vi "SRV_PM_Data Byte Unstuffing.vi"(0 "Stuffed Data":u8[](array[numeric]) format="%.0x", 1 "Data Length":u32, 11 "error in (no error)":errorcluster) -> (4 "Stuffed Data dup":u8[](array[numeric]) format="%.0x", 8 "Data":u8[](array[numeric]) format="%.0x", 10 "All Data Received?":bool, 14 "Remaining Stuffed Data":u8[](array[numeric]) format="%.0x", 15 "error out":errorcluster)   [LabVIEW 2009]
panel:
  in  "Stuffing Byte (0x00)":u8 format="%.0x"
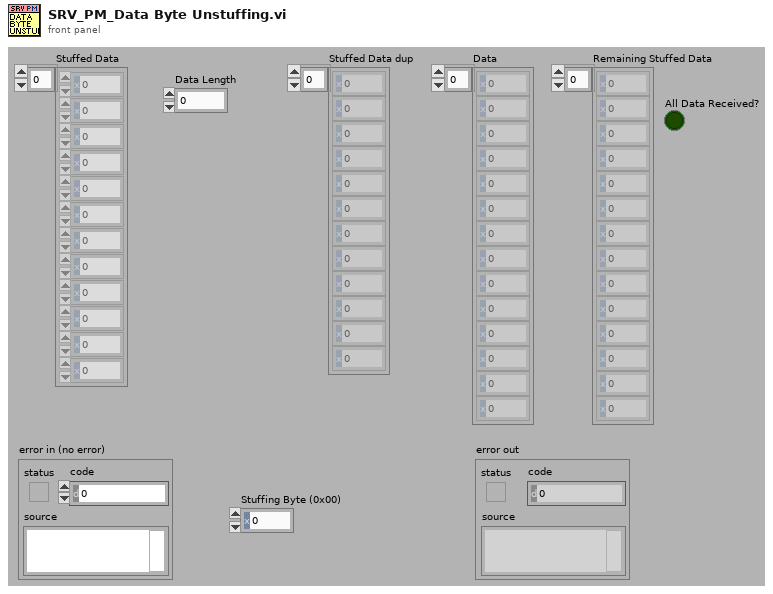
[diagram p1: front panel]
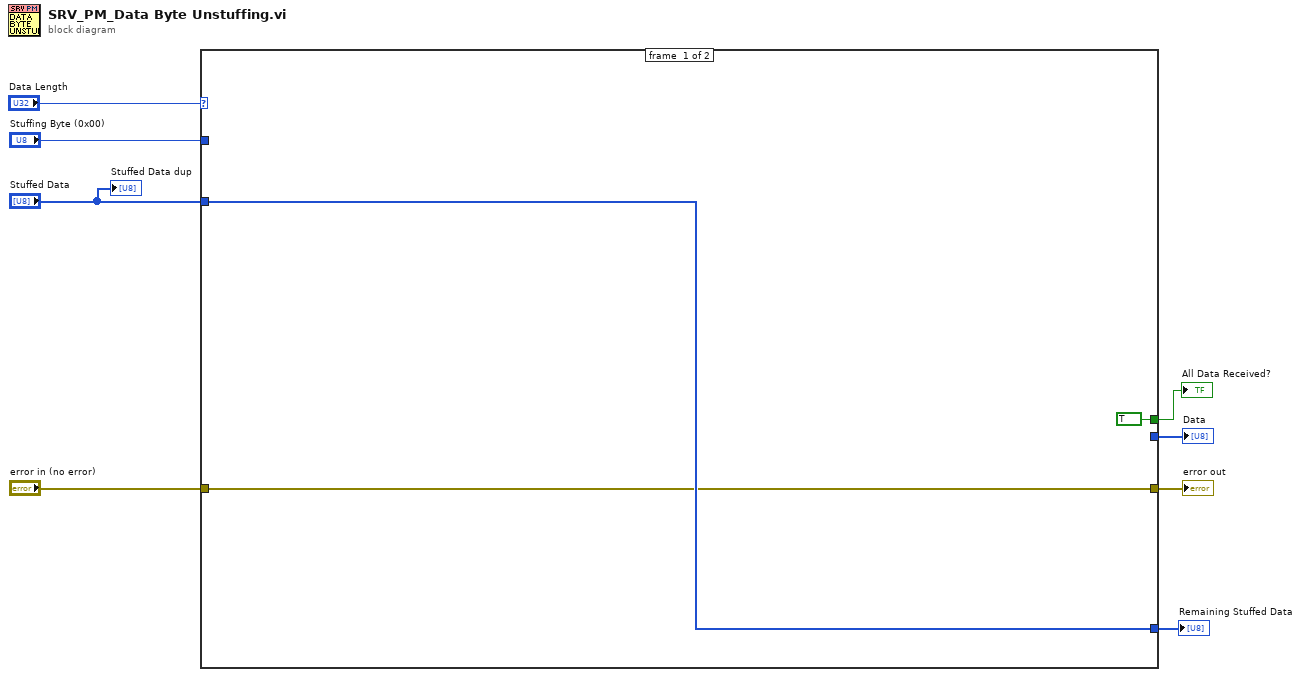
[diagram p0: block diagram]
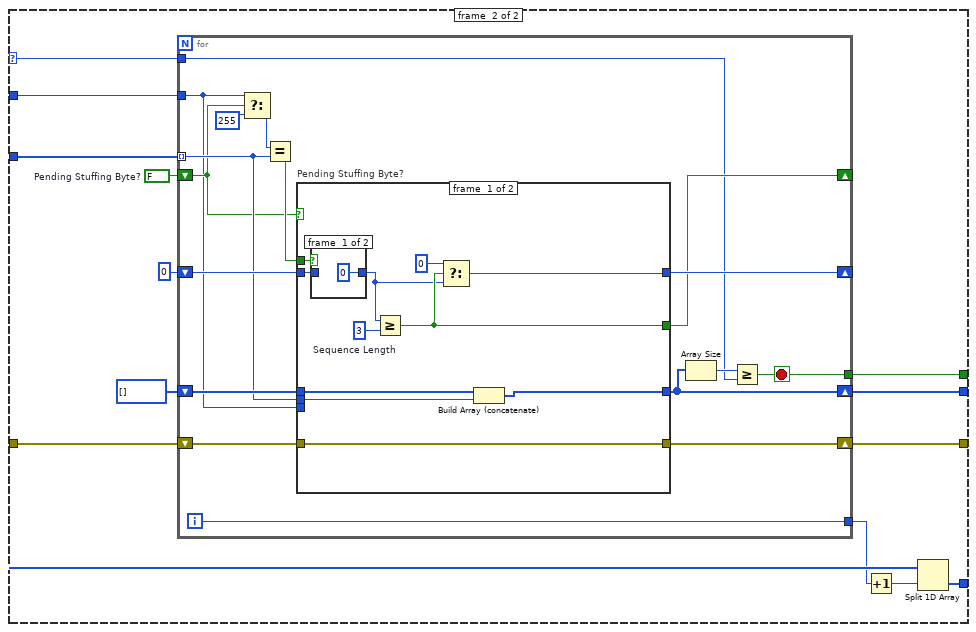
[diagram p2: hidden frame]
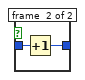
[diagram p3: hidden frame]
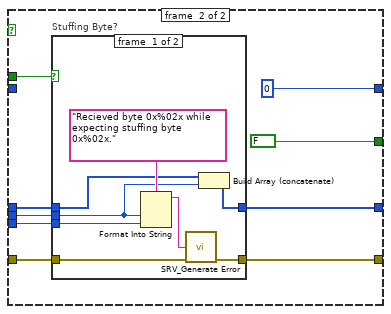
[diagram p4: hidden frame]
diagram:
  n1 = case shown="Default" "Data Length" {
    selector: "Data Length" -> [_ w13]
    tunnel: [_ w22] -> w8
    tunnel: "Stuffing Byte (0x00)" -> [_ w20]
    tunnel: "error in (no error)" -> [w10 w19]
    tunnel: [w10 w18] -> w5
    tunnel: "Stuffed Data" -> [w11 w17]
    tunnel: [w11 w15] -> w3
    tunnel: [TRUE w12] -> w1
    frame #0 {
    }
    frame #1 {
      w21 = FALSE  # Pending Stuffing Byte?
      n2 = for {
        tunnel: w17 -> [w37] mode=indexing
        shift-right: [w39] -> _
        shift-left: 0 -> [w40]
        shift-right: [w29] -> w22
        shift-left: u8[] [] ("Stuffed Data") -> [w38]
        shift-right: [w36] -> _
        shift-left: w21 -> [w33]
        tunnel: w20 -> [w30]
        shift-right: [w31] -> w18
        shift-left: w19 -> [w32]
        tunnel: w13 -> [w27]
        tunnel: [w26] -> w16
        tunnel: [w25] -> w12
        i -> [w26]
        stop <- w25 stop-if-true
        n3 = Select(t=w30, s=w33, f=u8 255) -> (s? t:f=w34:u8)
        n4 = Equal?(x=w34, y=w37) -> (x = y?=w41:bool)
        n5 = case "Pending Stuffing Byte?" shown="False" w33 {
          tunnel: w41 -> [w52 w64]
          tunnel: w40 -> [w51 _]
          tunnel: [w43 0] -> w39
          tunnel: w38 -> [w49 w63]
          tunnel: [w48 w62] -> w29
          tunnel: w37 -> [w47 w57]
          tunnel: [w46 FALSE] -> w36
          tunnel: w32 -> [w42 w59]
          tunnel: [w42 w58] -> w31
          tunnel: w30 -> [_ w56]
          frame #0 {
            w50 = 3  # Sequence Length
            n6 = case shown="True" w52 {
              tunnel: w51 -> [_ w55]
              tunnel: [0 w54] -> w44
              frame #0 {
              }
              frame #1 {
                n7 = Increment(x=w55) -> (x+1=w54:i32)
              }
            }
            n8 = Greater Or Equal?(x=w44, y=w50) -> (x >= y?=w46:bool)
            n9 = Select(t=0, s=w46, f=w44) -> (s? t:f=w43:i32)
            n10 = Build Array (concatenate)(w49, w47) -> (w48:u8[])
          }
          frame #1 {
            n11 = case "Stuffing Byte?" shown="False" w64 {
              tunnel: w63 -> [w66 w74]
              tunnel: [w67 w74] -> w62
              tunnel: w59 -> [w72 w73]
              tunnel: [w71 w73] -> w58
              tunnel: w57 -> [w65 _]
              tunnel: w56 -> [w69 _]
              frame #0 {
                n12 = Format Into String(format string="Recieved byte 0x%02x while expecting stuffing byte 0x%02x.", w65, w69) -> (resulting string=w70:string)  [unwired: 2 in, 1 out]
                n13 = call "SRV_Generate Error.vi"("Message"=w70, "error in (no error)"=w72) -> ("error out"=w71:errorcluster)  [unwired: 13 in]
                n14 = Build Array (concatenate)(w66, w65) -> (w67:u8[])
              }
              frame #1 {
              }
            }
          }
        }
        n15 = Array Size(array=w29) -> (size(s)=w28:i32)
        n16 = Greater Or Equal?(x=w28, y=w27) -> (x >= y?=w25:bool)
      }
      n17 = Increment(x=w16) -> (x+1=w14:i32)
      n18 = Split 1D Array(array=w17, index=w14) -> (second subarray=w15:u8[])  [unwired: 1 out]
    }
  }
  "error out" <- w5
  "Data" <- w8
  "Remaining Stuffed Data" <- w3
  "All Data Received?" <- w1
  "Stuffed Data dup" <- "Stuffed Data"
